vi "JEN.vi"(0 "System no.":i32=1 min=1 max=4 step=1, 3 "Joystick control":bool=TRUE, 5 "error in":errorcluster) -> (19 "error out":errorcluster)   [LabVIEW 2020]
doc: "Switches controller joystick control on (TRUE) or off (FALSE). Before using a joystick connected to the C-848 controller, calibrate joystick by running PI Terminal.vi. Type \"JEN CALIB\" and follow the instructions on the screen. \nSettings will not influence Joystick_Operation_Sample_Program.vi which works with a joystick connected to the host computer."
panel:
  # "Switches joystick control on (TRUE) or off (FALSE)."
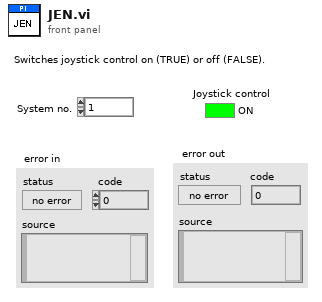
[diagram p1: front panel]
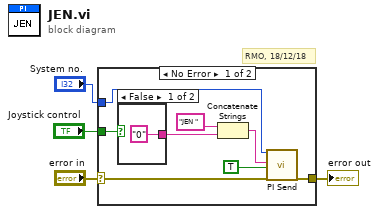
[diagram p0: block diagram]
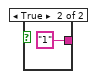
[diagram p2: hidden frame]
diagram:
  # "RMO, 18/12/18"
  n1 = case shown="No Error" "error in" {
    selector: "error in" -> [w5 w15]
    tunnel: "System no." -> [w10 _]
    tunnel: "Joystick control" -> [w8 _]
    tunnel: [w6 w15] -> w2
    frame No Error {
      n2 = case shown="False" w8 {
        tunnel: ["0" "1"] -> w7
        frame False {
        }
        frame True {
        }
      }
      n3 = Concatenate Strings("JEN ", w7) -> (w9:string)
      n4 = call "PI Send.vi"("System no."=w10, "String to send"=w9, "Attach termination char.?"=TRUE ("Attach Linefeed?"), "error in"=w5) -> ("error out"=w6:errorcluster)  [unwired: 2 in, 13 out]
    }
    frame Error {
    }
  }
  "error out" <- w2
